vi "Get myRIO Devices.vi"(8 "error in":errorcluster, 9 "Supported Devices":u32[](array[numeric]), 10 "Operation":enum16{"Get PID via USB", "Get PID via WiFi"}(ring), 11 "OwningVI":refnum<vi>) -> (0 "error out":errorcluster, 2 "TargetList":string[](array[string]), 3 "Detected Targets Info":T1[](array[typedef]))   [LabVIEW 2021, in "myRIOMetaDataObj.lvclass"]
uses:
  myRIOMetaDataObj.lvclass
  <resource>/myRIO/Target Info.ctl
  <resource>/myRIO/Included NICs For Discovery.ctl
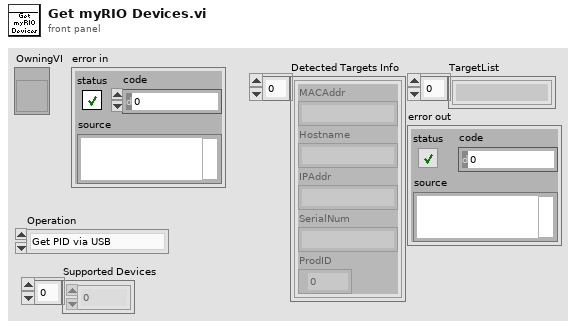
[diagram p1: front panel]
types:
  T1 = typedef "Target Info.ctl" = cluster{"MACAddr":string, "Hostname":string, "IPAddr":string, "SerialNum":string, "ProdID":u32}
  T2 = typedef "Included NICs For Discovery.ctl" = enum16{"All", "USBLAN only", "All but USBLAN"}
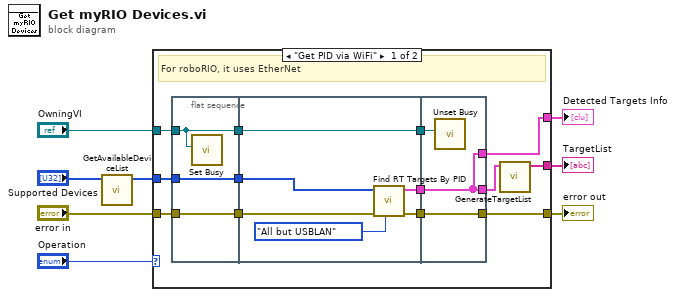
[diagram p0: block diagram]
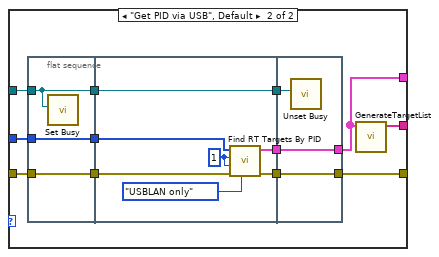
[diagram p2: hidden frame]
diagram:
  n1 = call "GetAvailableDeviceList.vi"("Supported Devices"="Supported Devices") -> ("Available Device List"=w1:u32[])  [unwired: 10 in]
  n2 = case shown="\"Get PID via WiFi\"" "Operation" {
    tunnel: "OwningVI" -> [w16 w40]
    tunnel: [w14 w39] -> w7
    tunnel: [w13 w38] -> w6
    tunnel: [w12 w37] -> w5
    tunnel: "error in" -> [w11 w36]
    tunnel: w1 -> [w10 w34]
    frame "Get PID via WiFi" {
      # "For roboRIO, it uses EtherNet"
      n3 = flat-sequence {
        tunnel: w16 -> [w24]
        tunnel: [w24] -> w21
        tunnel: w11 -> [w23]
        tunnel: [w23] -> w20
        tunnel: w10 -> [w22]
        tunnel: [w22] -> w9
        tunnel: [w30] -> w19
        tunnel: [w29] -> w18
        tunnel: [w28] -> w17
        tunnel: w21 -> [w28]
        tunnel: w20 -> [w27]
        tunnel: w9 -> [w25]
        tunnel: [w33] -> w12
        tunnel: [w31] -> w14
        tunnel: w19 -> [w31]
        tunnel: w18 -> [w33]
        tunnel: w17 -> [w32]
        tunnel: [w31] -> w15
        frame #0 {
          n4 = call <vilib>:"Set Busy.vi"("VI reference (current VI)"=w24) -> ()  [unwired: 9 in, 2 out]
        }
        frame #1 {
          n5 = call <resource>:"Find RT Targets By PID.vi"("Included NICs For Discovery"=Included_NICs_For_Discovery."All but USBLAN", "Error In"=w27, "PIDs To Discover"=w25) -> ("error out"=w29:errorcluster, "Detected Targets"=w30:T1[])  [unwired: 7 in]
        }
        frame #2 {
          n6 = call <vilib>:"Unset Busy.vi"("VI reference (current VI)"=w32) -> ()  [unwired: 10 in, 1 out]
        }
      }
      n7 = call "GenerateTargetList.vi"("Detected Targets"=w15) -> ("TargetList"=w13:string[])  [unwired: 10 in]
    }
    frame "Get PID via USB", Default {
      n8 = flat-sequence {
        tunnel: w40 -> [w48]
        tunnel: [w48] -> w45
        tunnel: w36 -> [w47]
        tunnel: [w47] -> w44
        tunnel: [w46] -> w35
        tunnel: w34 -> [w46]
        tunnel: [w55] -> w43
        tunnel: [w54] -> w42
        tunnel: [w53] -> w41
        tunnel: w45 -> [w53]
        tunnel: w44 -> [w52]
        tunnel: w35 -> [w49]
        tunnel: [w58] -> w37
        tunnel: w43 -> [w56]
        tunnel: w42 -> [w58]
        tunnel: w41 -> [w57]
        tunnel: [w56] -> w39
        frame #0 {
          n9 = call <vilib>:"Set Busy.vi"("VI reference (current VI)"=w48) -> ()  [unwired: 9 in, 2 out]
        }
        frame #1 {
          w50 = 1 ("Browse Timeout (sec)")
          n10 = call <resource>:"Find RT Targets By PID.vi"("Included NICs For Discovery"=Included_NICs_For_Discovery."USBLAN only", "Error In"=w52, "Resolve Timeout (sec)"=w50, "Browse Timeout (sec)"=w50, "PIDs To Discover"=w49) -> ("error out"=w54:errorcluster, "Detected Targets"=w55:T1[])  [unwired: 5 in]
        }
        frame #2 {
          n11 = call <vilib>:"Unset Busy.vi"("VI reference (current VI)"=w57) -> ()  [unwired: 10 in, 1 out]
        }
      }
      n12 = call "GenerateTargetList.vi"("Detected Targets"=w39) -> ("TargetList"=w38:string[])  [unwired: 10 in]
    }
  }
  "Detected Targets Info" <- w7
  "TargetList" <- w6
  "error out" <- w5
